vi "vectorField.vi"(4 "mostCoords":T1, 5 "thiccness":sgl, 6 "colourRampVals":cluster{"value":dbl, "colour":u32}[](array[cluster]), 7 "scale":dbl, 8 "error in (no error)":errorcluster, 9 "style":enum16{"Round", "Square"}(ring), 10 "vectorInfo":T2 {"UVW-TI" format="%#_3g"; "XYZ-WD" format="%#_4f"}, 11 "SceneObject in":refnum<vi>) -> (0 "error out":errorcluster, 3 "SceneObject out":refnum<vi>)   [LabVIEW 2022 SP3]
uses:
  vectorDef.ctl
  coordSys.ctl
  <vilib>/Analysis/coordinate.llb/3D Coordinate Conversion (Scalar).vi
  Anemometry/Anemometry Sub Vis/Data_plotting_vis/Results_plotter_Global.vi
  <vilib>/picture/3D Picture Control/Object/Create Object (drawable).vi
  <vilib>/picture/3D Picture Control/Object/Add Object (no reference).vi
  <vilib>/picture/3D Picture Control/NI_3D Picture Control.lvlib
  <vilib>/Analysis/NI_AALPro.lvlib
panel:
  in  "giveUp!":bool
  out "loop":i32
  out "Name":string
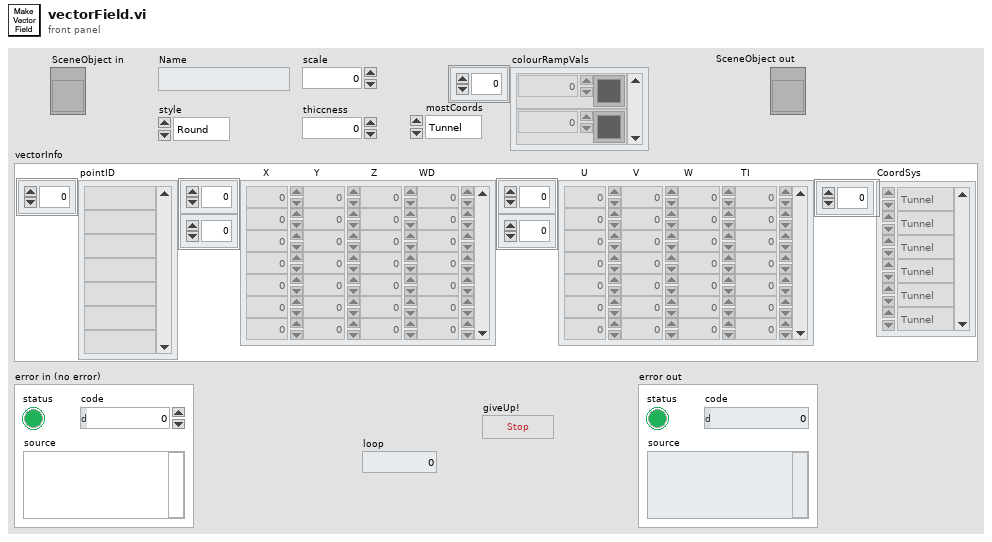
[diagram p1: front panel]
types:
  T1 = typedef "coordSys.ctl" = enum16{"Tunnel", "Model"}
  T2 = typedef "vectorDef.ctl" = cluster{"pointID":string[], "XYZ-WD":dbl[][], "UVW-TI":dbl[][], "CoordSys":T1[]}
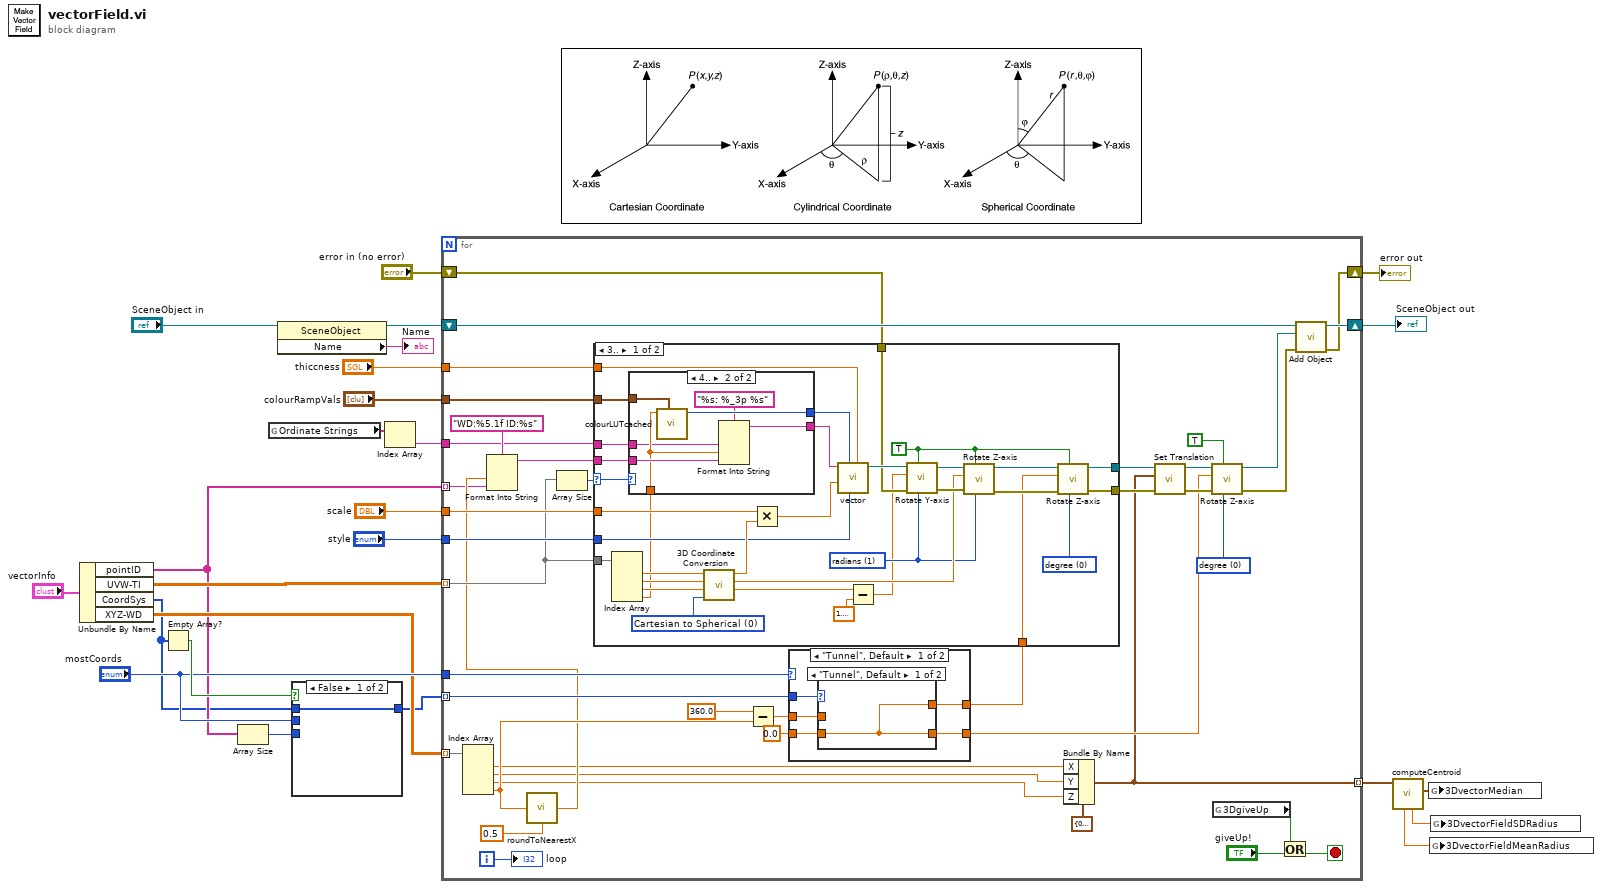
[diagram p0: block diagram]
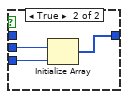
[diagram p2: hidden frame]
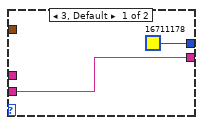
[diagram p6: hidden frame]
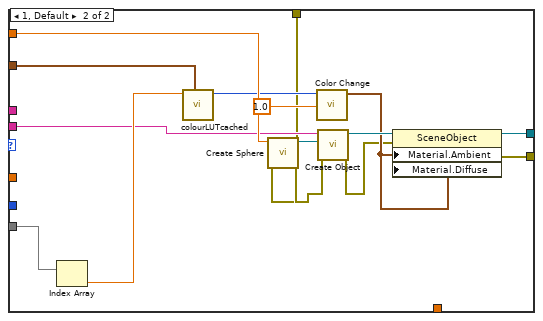
[diagram p7: hidden frame]
diagram:
  n1 = Unbundle By Name("vectorInfo") -> ("pointID"=w9:string[], "UVW-TI"=w15:dbl[][], "CoordSys"=w7:T1[], "XYZ-WD"=w11:dbl[][])
  n2 = Empty Array?(array=w7) -> (empty?=w13:bool)
  n3 = Array Size(array=w9) -> (size(s)=w10:i32)
  n4 = global read "Results_plotter_Global.vi" "Ordinate Strings"() -> (w6:string[])
  n5 = property class="SceneObject"(reference="SceneObject in") -> (reference out=w16:refnum<vi>, "Name"=→"Name":string)  [unwired: 1 in, 1 out]
  n6 = case shown="False" w13 {
    tunnel: "mostCoords" -> [_ w29]
    tunnel: w10 -> [_ w28]
    tunnel: [w26 w27] -> w8
    tunnel: w7 -> [w26 _]
    frame False {
    }
    frame True {
      n7 = Initialize Array(w29, w28) -> (w27:T1[])
    }
  }
  n8 = Index Array(array=w6) -> (element=w5:string)  [unwired: 1 in]
  n9 = for {
    shift-right: [w70] -> w17
    shift-left: w16 -> [w71]
    shift-right: [w69] -> w21
    shift-left: "error in (no error)" -> [w67]
    tunnel: "scale" -> [w66]
    tunnel: "thiccness" -> [w65]
    tunnel: "style" -> [w64]
    tunnel: w9 -> [w38] mode=indexing
    tunnel: w11 -> [w63] mode=indexing
    tunnel: w15 -> [w59] mode=indexing
    tunnel: "colourRampVals" -> [w60]
    tunnel: w8 -> [w45] mode=indexing
    tunnel: "mostCoords" -> [w46]
    tunnel: w5 -> [w40]
    tunnel: [w34] -> w4 mode=indexing
    i -> [w33]
    stop <- w31 stop-if-true
    w53 = u16 0 items=["degree", "radians"] ("angle unit")
    n10 = Index Array(array=w63) -> (element #1=w37:dbl, element #2=w36:dbl, element #3=w35:dbl, element #4=w55:dbl)  [unwired: 4 in]
    n11 = call "roundToNearestX.vi"("Numeric"=w55, "Round to Nearest"=0.5) -> ("roundNearest"=w39:dbl)  [unwired: 1 in, 1 out]
    n12 = Format Into String(format string="WD:%5.1f ID:%s", w39, w38) -> (resulting string=w57:string)  [unwired: 2 in, 1 out]
    n13 = Array Size(array=w59) -> (size(s)=w58:i32)
    n14 = Subtract(x=360.0, y=w55) -> (x-y=w43:dbl)
    n15 = case shown="\"Tunnel\", Default" w46 {
      tunnel: w45 -> [w76 w83]
      tunnel: [w75 w82] -> w44
      tunnel: w43 -> [w74 w81]
      tunnel: [w73 w80] -> w42
      tunnel: 0.0 -> [w72 w79]
      frame "Tunnel", Default {
        n16 = case shown="\"Tunnel\", Default" w76 {
          tunnel: [w77 w78] -> w75
          tunnel: w74 -> [_ w78]
          tunnel: [w77 w78] -> w73
          tunnel: w72 -> [w77 _]
          frame "Tunnel", Default {
          }
          frame "Model" {
          }
        }
      }
      frame "Model" {
        n17 = case shown="\"Tunnel\", Default" w83 {
          tunnel: [w84 w87] -> w82
          tunnel: w81 -> [w85 w87]
          tunnel: [w85 w86] -> w80
          tunnel: w79 -> [w84 w86]
          frame "Tunnel", Default {
          }
          frame "Model" {
          }
        }
      }
    }
    n18 = case shown="3.." w58 {
      selector: w58 -> [w93 _]
      tunnel: w67 -> [w109 w130]
      tunnel: w66 -> [w108 _]
      tunnel: w65 -> [w107 w139]
      tunnel: w64 -> [w106 _]
      tunnel: w57 -> [w89 w133]
      tunnel: w59 -> [w102 w144]
      tunnel: [w100 w134] -> w62
      tunnel: [w98 w135] -> w61
      tunnel: w60 -> [w95 w143]
      tunnel: w44 -> [w92 _]
      tunnel: w40 -> [w88 _]
      frame 3.. {
        w96 = u16 0 items=["degree", "radians"] ("angle unit")
        w111 = u16 1 items=["degree", "radians"] ("angle unit")
        w97 = TRUE ("Relative?")
        w116 = u16 0 items=["Cartesian to Spherical", "Spherical to Cartesian", "Cartesian to Cylindrical", "Cylindrical to Cartesian", "Spherical to Cylindrical", "Cylindrical to Spherical"] ("conversion type")
        n19 = Index Array(array=w102) -> (element #1=w119:dbl, element #2=w118:dbl, element #3=w117:dbl, element #4=w91:dbl)  [unwired: 4 in]
        n20 = case shown="4.." w93 {
          tunnel: w95 -> [_ w129]
          tunnel: w91 -> [_ w124]
          tunnel: [u32 16711178 ("colour") w128] -> w94
          tunnel: [w121 w126] -> w90
          tunnel: w89 -> [w121 w125]
          tunnel: w88 -> [_ w123]
          frame 3, Default {
          }
          frame 4.. {
            n21 = call "colourLUTcached.vi"("rampMarkers"=w129, "value"=w124) -> ("colour"=w128:u32)  [unwired: 7 in, 2 out]
            n22 = Format Into String(format string="%s: %_3p %s", w123, w124, w125) -> (resulting string=w126:string)  [unwired: 2 in, 1 out]
          }
        }
        n23 = call-poly <vilib>:"3D Coordinate Conversion.vi"("conversion type"=w116, "axis 3"=w117, "axis 2"=w118, "axis 1"=w119) -> ("axis 3 out"=w105:dbl, "axis 2 out"=w112:dbl, "axis 1 out"=w115:dbl)  [unwired: 4 in, 1 out]
        n24 = Multiply(x=w108, y=w115) -> (x*y=w120:dbl)
        n25 = call "vector.vi"("thiccness"=w107, "style"=w106, "Color"=w94, "Length X"=w120, "Name"=w90) -> ("SceneObject out"=w110:refnum<vi>)  [unwired: 5 in, 1 out]
        n26 = Subtract(x=w105, y=1.5707963267948966) -> (x-y=w103:dbl)
        n27 = call <vilib>:"Rotate Y-axis.vi"("angle unit"=w111, "Relative?"=w97, "error in (no error)"=w109, "angle"=w103, "Scene Object In"=w110) -> ("error out"=w114:errorcluster, "Scene Object Out"=w113:refnum<vi>)  [unwired: 5 in]
        n28 = call <vilib>:"Rotate Z-axis.vi"("angle unit"=w111, "Relative?"=w97, "error in (no error)"=w114, "angle"=w112, "Scene Object In"=w113) -> ("error out"=w101:errorcluster, "Scene Object Out"=w99:refnum<vi>)  [unwired: 5 in]
        n29 = call <vilib>:"Rotate Z-axis.vi"("angle unit"=w96, "Relative?"=w97, "error in (no error)"=w101, "angle"=w92, "Scene Object In"=w99) -> ("error out"=w100:errorcluster, "Scene Object Out"=w98:refnum<vi>)  [unwired: 5 in]
      }
      frame 1, Default {
        n30 = Index Array(array=w144) -> (element=w142:dbl)  [unwired: 1 in]
        n31 = call "colourLUTcached.vi"("rampMarkers"=w143, "value"=w142) -> ("colour"=w136:u32)  [unwired: 7 in, 2 out]
        n32 = call <vilib>:"Create Sphere.vi"("error in (no error)"=w130, "Radius"=w139) -> ("error out"=w132:errorcluster, "New Sphere Refnum"=w140:refnum<vi>)  [unwired: 8 in]
        n33 = call <vilib>:"Color Change.vi"("Alpha"=1.0, "Color"=w136) -> ("RGBA"=w137:cluster{"R":sgl, "G":sgl, "B":sgl, "A":sgl})  [unwired: 9 in]
        n34 = call-poly <vilib>:"Create Object.vi"("error in (no error)"=w132, "Geometry"=w140, "Name"=w133) -> ("error out"=w131:errorcluster, "Scene:New Object"=w138:refnum<vi>)  [unwired: 7 in]
        n35 = property class="SceneObject"(reference=w138, error in=w131, "Material.Ambient"=w137, "Material.Diffuse"=w137) -> (reference out=w135:refnum<vi>, error out=w134:errorcluster)
      }
    }
    n36 = Bundle By Name(cluster=cluster{"X":sgl, "Y":sgl, "Z":sgl} {"X"=0.0, "Y"=0.0, "Z"=0.0} ("Translation"), "X"=w37, "Y"=w36, "Z"=w35) -> (w34:cluster{"X":sgl, "Y":sgl, "Z":sgl})
    n37 = call <vilib>:"Set Translation.vi"("error in (no error)"=w62, "Translation"=w34, "Scene Object"=w61) -> ("error out"=w52:errorcluster, "Translated Object"=w51:refnum<vi>)  [unwired: 7 in]
    n38 = call <vilib>:"Rotate Z-axis.vi"("angle unit"=w53, "Relative?"=TRUE, "error in (no error)"=w52, "angle"=w42, "Scene Object In"=w51) -> ("error out"=w49:errorcluster, "Scene Object Out"=w50:refnum<vi>)  [unwired: 5 in]
    n39 = global read "Results_plotter_Global.vi" "3DgiveUp"() -> (w30:bool)
    n40 = Or(x=w30, y="giveUp!") -> (x .or. y?=w31:bool)
    n41 = call-poly <vilib>:"Add Object.vi"("error in (no error)"=w49, "New Object In"=w50, "Scene Object In"=w71) -> ("error out"=w69:errorcluster, "Scene Object Out"=w70:refnum<vi>)  [unwired: 7 in]
    "loop" <- w33
  }
  "error out" <- w21
  "SceneObject out" <- w17
  n42 = call "computeCentroid.vi"("locations"=w4) -> ("median"=w3:cluster{"X":sgl, "Y":sgl, "Z":sgl}, "SDradius"=w2:dbl, "meanRadius"=w1:dbl)  [unwired: 8 in]
  n43 = global write "Results_plotter_Global.vi" "3DvectorMedian"(w3) -> ()
  n44 = global write "Results_plotter_Global.vi" "3DvectorFieldMeanRadius"(w1) -> ()
  n45 = global write "Results_plotter_Global.vi" "3DvectorFieldSDRadius"(w2) -> ()
